vi "Calibration and Update Routine.vi"(8 "simTC Channels":dbl[](array[numeric])=[102.0], 9 "Cal Channels":dbl[](array[numeric])=[25.0, 0.0, 703.6], 10 "TC Update State":T1=enum."Update", 11 "RT Configuration Data":T2={"Current Task"="", "Voltage Task"="", "FIFO Sort Key"=[], "Cal Channel Indicies"=[0, 255, 255, 255, 255, 255, 255, 255], "Current Initial Values"=[], "Voltage Initial Values"=[], "TC Channel Config"=[{"Thermocouple Type"=0, "Temperature Units"=0}], "TC Update Period"=0.0, "Voltage Divider Ratio"=0.099, "Samples To Collect"=25.0, "Temperature Units"=0, "Cal Settling Time"=1.0, "Cal Types"=[0]} {"Cal Types" items=["J", "K", "T", "E", "N", "B", "R", "S"]; "Temperature Units" items=["Celcius", "Fahrenheit", "Kelvin", "Rankine"]; "TC Channel Config"."Temperature Units" items=["Celcius", "Fahrenheit", "Kelvin", "Rankine", "Volts"]; "TC Channel Config"."Thermocouple Type" items=["J", "K", "T", "E", "N", "B", "R", "S", "Raw Voltage"]}) -> (1 "Cal Valid?":bool, 2 "Error":dbl[](array[numeric])=[-2.86286859433152], 3 "Voltages to Output":dbl[](array[numeric])=[0.0003896684])   [LabVIEW 2011, in "Simulated Thermocouple Custom Device.lvlib"]
uses:
  Simulated Thermocouple Custom Device.lvlib
  RT Config Data.ctl
  TC Channel Config Data.ctl
  TC Selector.ctl
  TC Unit Selector.ctl
  RT TC Update State.ctl
panel:
  out "Desired temperatures to output (for debug)":dbl[](array[numeric])
  out "Reset Cal Flag":bool=TRUE
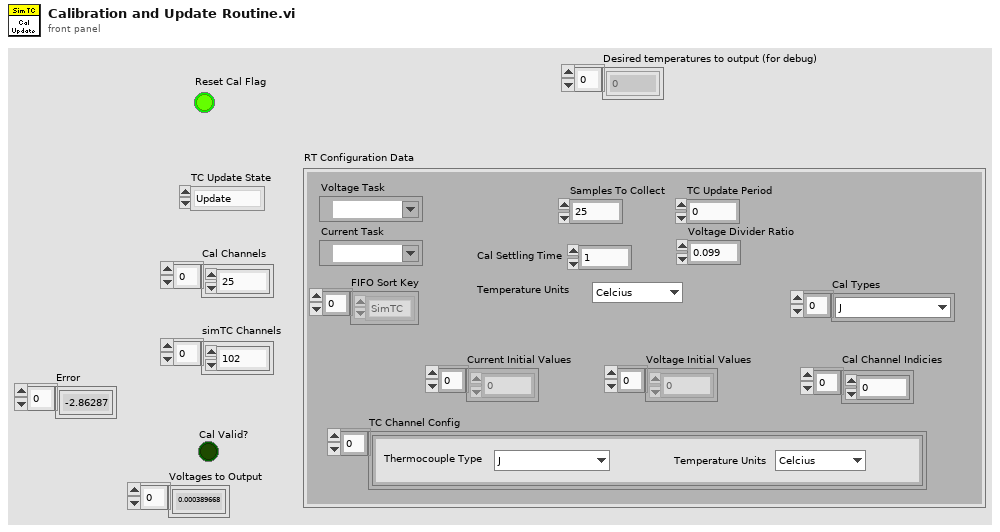
[diagram p1: front panel]
types:
  T1 = typedef "Simulated Thermocouple Custom Device.lvlib/RT TC Update State.ctl" = enum16{"Init", "Calibrate", "Update", "Idle"}
  T2 = typedef "Simulated Thermocouple Custom Device.lvlib/RT Config Data.ctl" = cluster{"Current Task":refnum<k21>, "Voltage Task":refnum<k21>, "FIFO Sort Key":enum16{"SimTC", "Calibration", "VO", "CO"}[], "Cal Channel Indicies":i32[], "Current Initial Values":dbl[], "Voltage Initial Values":dbl[], "TC Channel Config":T3[], "TC Update Period":dbl, "Voltage Divider Ratio":dbl, "Samples To Collect":dbl, "Temperature Units":T5, "Cal Settling Time":dbl, "Cal Types":T4[]}
  T3 = typedef "Simulated Thermocouple Custom Device.lvlib/TC Channel Config Data.ctl" = cluster{"Thermocouple Type":T4, "Temperature Units":T5}
  T4 = typedef "Simulated Thermocouple Custom Device.lvlib/TC Selector.ctl" = u16
  T5 = typedef "Simulated Thermocouple Custom Device.lvlib/TC Unit Selector.ctl" = u16
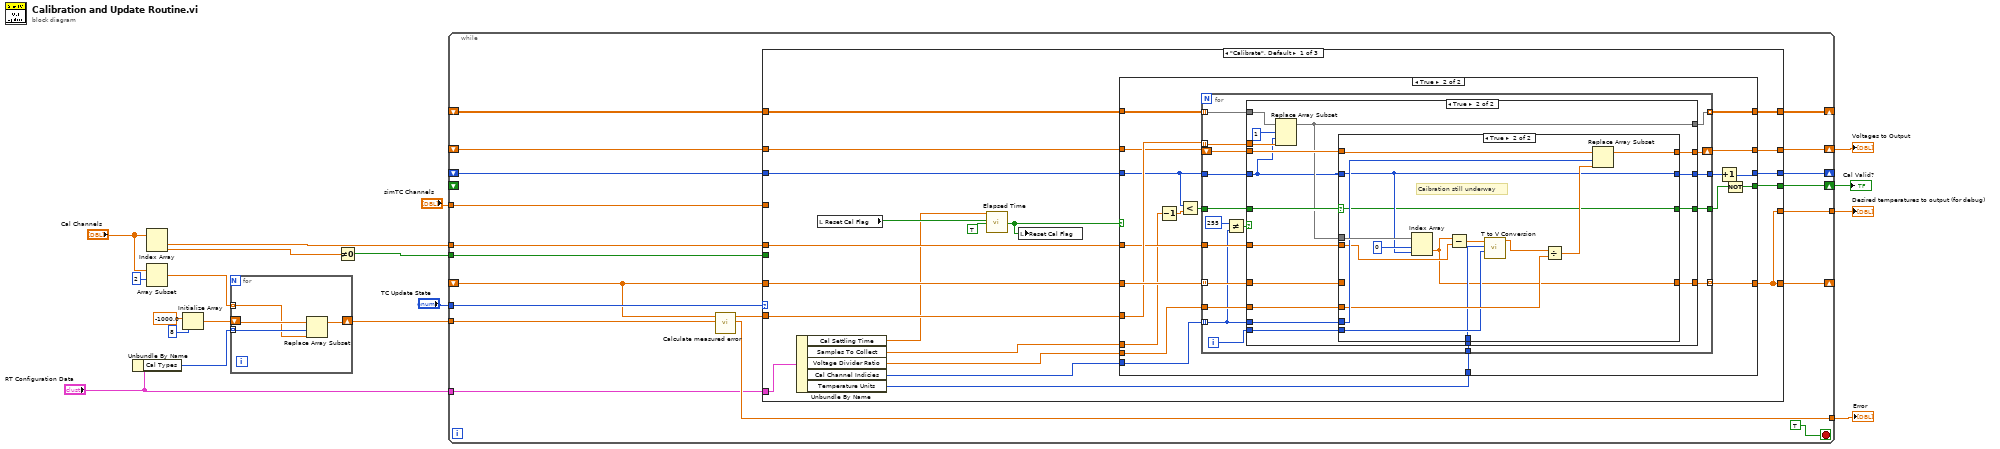
[diagram p0: block diagram]
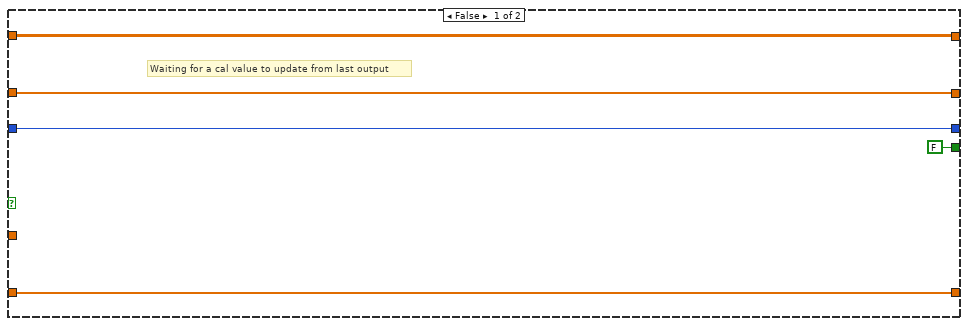
[diagram p2: hidden frame]
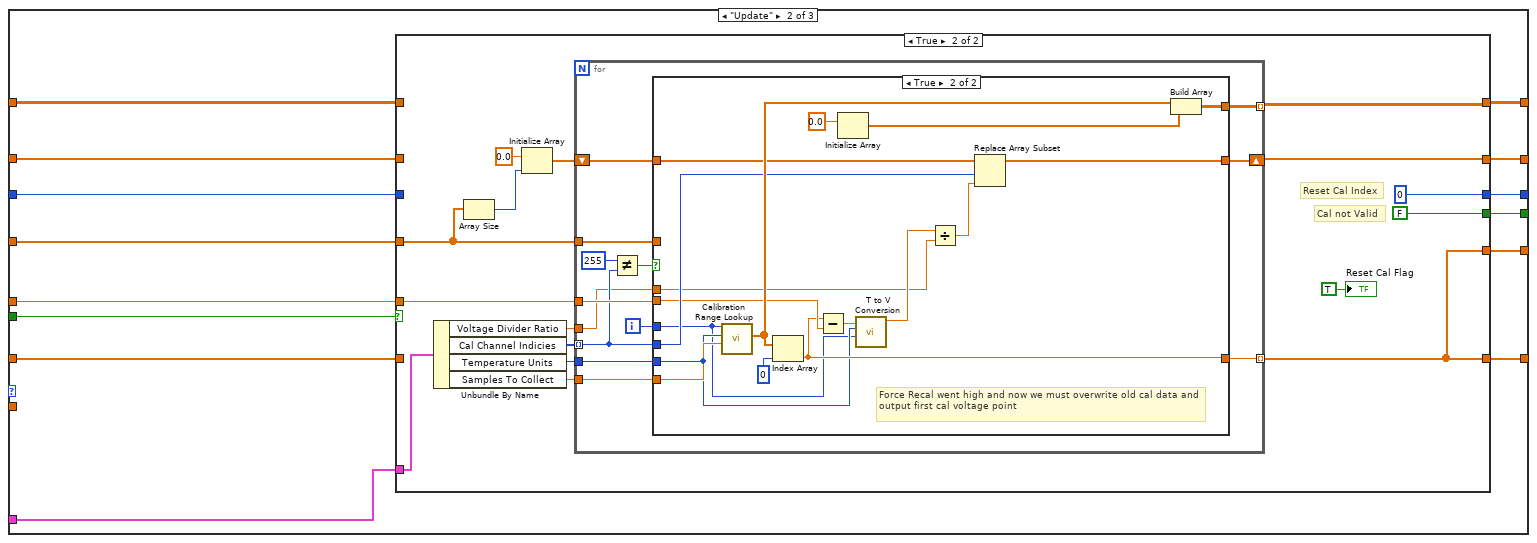
[diagram p5: hidden frame]
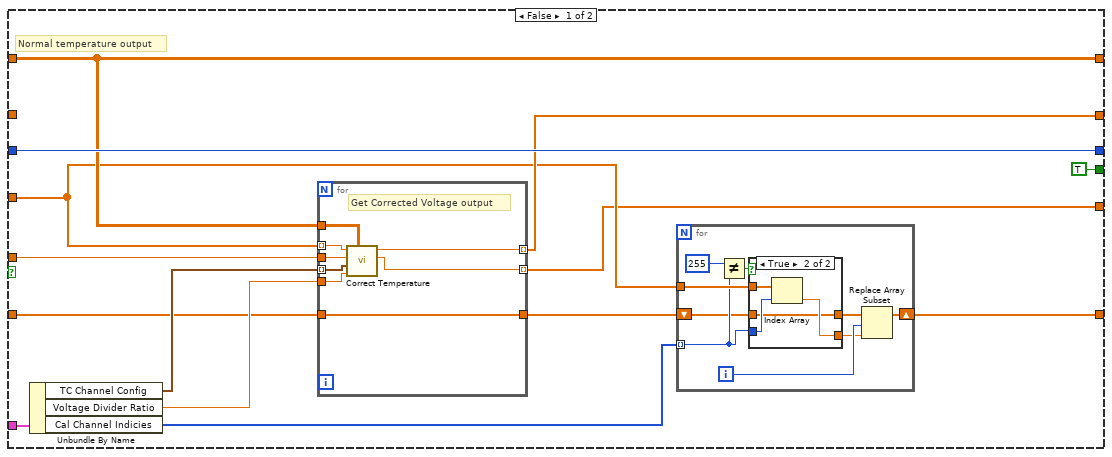
[diagram p6: hidden frame]
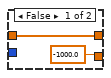
[diagram p7: hidden frame]
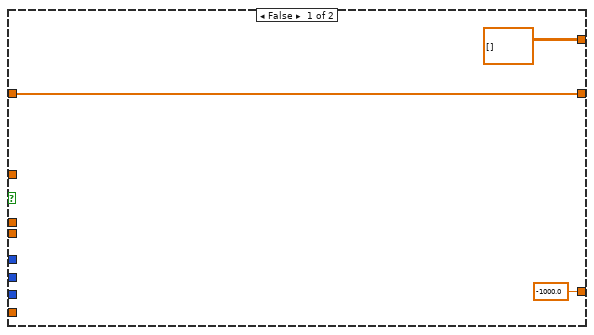
[diagram p8: hidden frame]
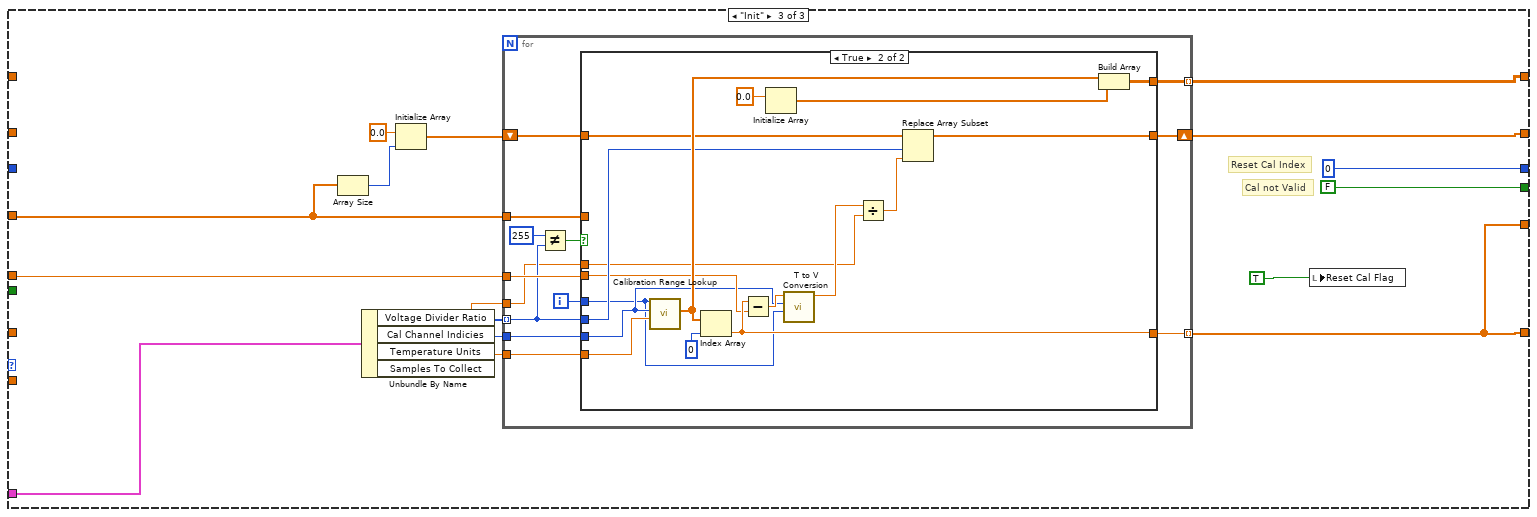
[diagram p9: hidden frame]
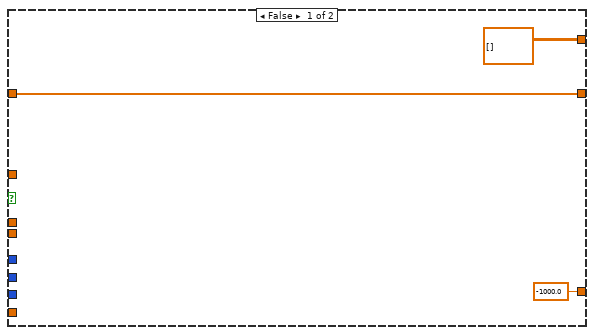
[diagram p10: hidden frame]
diagram:
  n1 = Unbundle By Name("RT Configuration Data") -> ("Cal Types"=w5:T4[])
  n2 = Index Array(array="Cal Channels") -> (element #1=w13:dbl, element #2=w12:dbl)  [unwired: 2 in]
  n3 = Array Subset(array="Cal Channels", index=2) -> (w9:dbl[])  [unwired: 1 in]
  n4 = Initialize Array(-1000.0 ("element"), 8 ("dimension size")) -> (w6:dbl[])
  n5 = for {
    tunnel: w9 -> [w19] mode=indexing
    shift-right: [w22] -> w4
    shift-left: w6 -> [w21]
    tunnel: w5 -> [w20] mode=indexing
    n6 = Replace Array Subset(array=w21, new element=w19, index=w20) -> (w22:dbl[])
  }
  n7 = Not Equal To 0?(x=w12) -> (x != 0?=w17:bool)
  n8 = while {
    tunnel: "TC Update State" -> [w40]
    tunnel: w4 -> [w26]
    tunnel: w13 -> [w28]
    tunnel: w17 -> [w37]
    shift-right: [w29] -> _
    shift-left: _ -> [w24]
    tunnel: "RT Configuration Data" -> [w30]
    shift-right: [w39] -> _
    shift-left: _ -> [w25]
    tunnel: "simTC Channels" -> [w38]
    shift-right: [w31] -> w2
    shift-left: _ -> [w34]
    tunnel: [w32] -> w15
    shift-right: [w36] -> _
    shift-left: _ -> [w27]
    shift-right: [w35] -> w14
    shift-left: _ -> [_]
    tunnel: [w23] -> w3
    stop <- TRUE stop-if-true
    n9 = call "Calculate measured error.vi"("> Cal Channel Value >"=w26, "Last Cal Channel Voltage Outputted"=w24) -> ("Error"=w32:dbl[], "Measured-Desired"=w33:dbl[])  [unwired: 8 in]
    n10 = case shown="\"Calibrate\", Default" w40 {
      tunnel: [w60 w158 w254] -> w39
      tunnel: w38 -> [_ w148 w245]
      tunnel: w25 -> [w61 w157 _]
      tunnel: w28 -> [w55 w156 w255]
      tunnel: w37 -> [_ w155 _]
      tunnel: w27 -> [w47 w152 _]
      tunnel: w33 -> [w58 _ _]
      tunnel: w24 -> [w46 w146 _]
      tunnel: [w59 w153 0] -> w36
      tunnel: [w57 w154 FALSE] -> w35
      tunnel: w34 -> [w56 w151 _]
      tunnel: [w48 w150 w253] -> w31
      tunnel: w30 -> [w51 w149 w256]
      tunnel: [w43 w147 w249] -> w29
      tunnel: [w43 w145 w249] -> w23
      frame "Calibrate", Default {
        n11 = Unbundle By Name(w51) -> ("Cal Settling Time"=w45:dbl, "Samples To Collect"=w50:dbl, "Voltage Divider Ratio"=w49:dbl, "Cal Channel Indicies"=w42:i32[], "Temperature Units"=w44:T5)
        n12 = local read "Reset Cal Flag"() -> (w53:bool)
        n13 = call "Elapsed Time"("Time Target (s)"=w45, "Reset"=w53, "Auto Reset"=TRUE) -> ("Time has Elapsed"=w52:bool)  [unwired: 9 in, 7 out]
        n14 = local write "Reset Cal Flag"(w52) -> ()
        n15 = case shown="True" w52 {
          tunnel: w61 -> [w65 w85]
          tunnel: [w65 w76] -> w60
          tunnel: w47 -> [w64 w77]
          tunnel: w46 -> [w62 w83]
          tunnel: [w64 w69] -> w59
          tunnel: w58 -> [_ w82]
          tunnel: [FALSE w68] -> w57
          tunnel: [w66 w80] -> w48
          tunnel: w56 -> [w66 w79]
          tunnel: w55 -> [_ w78]
          tunnel: w50 -> [_ w75]
          tunnel: w42 -> [_ w74]
          tunnel: w49 -> [_ w73]
          tunnel: [w62 w72] -> w43
          tunnel: w44 -> [_ w71]
          frame False {
            # "Waiting for a cal value to update from last output"
          }
          frame True {
            n16 = Decrement(x=w75) -> (x-1=w81:dbl)
            n17 = Less?(x=w77, y=w81) -> (x < y?=w84:bool)
            n18 = for {
              tunnel: w85 -> [w103] mode=indexing
              tunnel: w84 -> [w102]
              tunnel: [w101] -> w70
              tunnel: w83 -> [w100] mode=indexing
              tunnel: w82 -> [w99] mode=indexing
              tunnel: w78 -> [w96]
              tunnel: w77 -> [w92]
              tunnel: [w95] -> w76 mode=indexing
              tunnel: w74 -> [w90] mode=indexing
              tunnel: w73 -> [w94]
              tunnel: [w93] -> w72 mode=indexing
              tunnel: w71 -> [w87]
              tunnel: [w86] -> w67
              shift-right: [w98] -> w80
              shift-left: w79 -> [w97]
              i -> [w88]
              n19 = Not Equal?(x=255, y=w90) -> (x != y?=w91:bool)
              n20 = case shown="True" w91 {
                tunnel: w103 -> [w108 w125]
                tunnel: w102 -> [w104 w124]
                tunnel: [w106 w123] -> w101
                tunnel: w100 -> [w105 w122]
                tunnel: w99 -> [_ w121]
                tunnel: [w107 w120] -> w98
                tunnel: w97 -> [w107 w119]
                tunnel: w96 -> [_ w118]
                tunnel: [w108 w117] -> w95
                tunnel: w90 -> [_ w116]
                tunnel: w94 -> [_ w115]
                tunnel: [w105 w114] -> w93
                tunnel: w92 -> [w106 w112]
                tunnel: w88 -> [_ w111]
                tunnel: w87 -> [_ w110]
                tunnel: [w104 w109] -> w86
                frame False {
                }
                frame True {
                  n21 = Replace Array Subset(array=w125, new element=w121, index (row)=1 ("disabled index (row)"), index (col)=w112) -> (w117:dbl[][])
                  n22 = case shown="True" w124 {
                    selector: w124 -> [w126 w133]
                    tunnel: w112 -> [w129 w134]
                    tunnel: [w129 w134] -> w123
                    tunnel: w122 -> [w127 _]
                    tunnel: [w128 w143] -> w120
                    tunnel: w119 -> [w128 w141]
                    tunnel: w118 -> [_ w131]
                    tunnel: w117 -> [_ w142]
                    tunnel: w116 -> [_ w140]
                    tunnel: w115 -> [_ w138]
                    tunnel: [w127 w130] -> w114
                    tunnel: w111 -> [_ w136]
                    tunnel: w110 -> [_ w135]
                    tunnel: [w126 w133] -> w109
                    frame False {
                      # "Cal is Valid"
                      # "Last Step of Calibration completed"
                    }
                    frame True {
                      # "Caibration still underway"
                      n23 = Index Array(array=w142, index (row)=0, index (col)=w134) -> (element=w130:dbl)
                      n24 = Subtract(x=w130, y=w131) -> (x-y=w132:dbl)
                      n25 = call "T to V Conversion.vi"("Thermocouple Type"=w136, "Temperature Units"=w135, "Temperature"=w132) -> ("Voltage Out"=w137:dbl)  [unwired: 8 in]
                      n26 = Divide(x=w137, y=w138) -> (x/y=w139:dbl)
                      n27 = Replace Array Subset(array=w141, new element=w139, index=w140) -> (w143:dbl[])
                    }
                  }
                }
              }
            }
            n28 = Increment(x=w70) -> (x+1=w69:i32)
            n29 = Not(x=w67) -> (.not. x?=w68:bool)
          }
        }
      }
      frame "Update" {
        n30 = case shown="True" w155 {
          tunnel: [w166 w202] -> w158
          tunnel: w157 -> [w166 _]
          tunnel: w156 -> [w172 w204]
          tunnel: [TRUE FALSE] -> w154
          tunnel: [w171 0] -> w153
          tunnel: w152 -> [w171 _]
          tunnel: w151 -> [_ _]
          tunnel: [w169 w207] -> w150
          tunnel: w149 -> [w170 w209]
          tunnel: w148 -> [w160 w199]
          tunnel: [w162 w200] -> w147
          tunnel: w146 -> [w165 _]
          tunnel: [w159 w200] -> w145
          frame False {
            # "Normal temperature output"
            n31 = Unbundle By Name(w170) -> ("TC Channel Config"=w168:T3[], "Voltage Divider Ratio"=w167:dbl, "Cal Channel Indicies"=w164:i32[])
            n32 = for {
              tunnel: [w191] -> w169 mode=indexing
              tunnel: w172 -> [w195]
              tunnel: w160 -> [w189] mode=indexing
              tunnel: w168 -> [w194] mode=indexing
              tunnel: w167 -> [w193]
              tunnel: w166 -> [w192]
              tunnel: w165 -> [w190]
              tunnel: [w190] -> w163
              tunnel: [w188] -> w159 mode=indexing
              # "Get Corrected Voltage output"
              n33 = call "Correct Temperature.vi"("Cal LUT"=w192, "Divider Ratio"=w193, "TC Channel Config"=w194, "CJC"=w195, "Rquested Output Temp"=w189) -> ("Corrected Output Temp"=w188:dbl, "Voltage Out"=w191:dbl)  [unwired: 5 in]
            }
            n34 = for {
              tunnel: w164 -> [w176] mode=indexing
              tunnel: w160 -> [w181]
              shift-right: [w180] -> w162
              shift-left: w163 -> [w174]
              i -> [w179]
              n35 = Not Equal?(x=255, y=w176) -> (x != y?=w177:bool)
              n36 = case shown="True" w177 {
                tunnel: w181 -> [_ w187]
                tunnel: w176 -> [_ w186]
                tunnel: [-1000.0 ("Corrected Output Temp") w185] -> w178
                tunnel: w174 -> [w182 w184]
                tunnel: [w182 w184] -> w173
                frame False {
                }
                frame True {
                  n37 = Index Array(array=w187, index=w186) -> (element=w185:dbl)
                }
              }
              n38 = Replace Array Subset(array=w173, new element=w178, index=w179) -> (w180:dbl[])
            }
          }
          frame True {
            # "Cal not Valid"
            # "Reset Cal Index"
            n39 = Unbundle By Name(w209) -> ("Voltage Divider Ratio"=w201:dbl, "Cal Channel Indicies"=w206:i32[], "Temperature Units"=w208:T5, "Samples To Collect"=w203:dbl)
            n40 = Array Size(array=w199) -> (size(s)=w197:i32)
            n41 = Initialize Array(0.0 ("element"), w197) -> (w198:dbl[])
            n42 = for {
              tunnel: w208 -> [w224]
              tunnel: w199 -> [w223]
              tunnel: [w221] -> w200 mode=indexing
              tunnel: w206 -> [w217] mode=indexing
              tunnel: w204 -> [w220]
              tunnel: w203 -> [w219]
              tunnel: [w214] -> w202 mode=indexing
              tunnel: w201 -> [w212]
              shift-right: [w222] -> w207
              shift-left: w198 -> [w213]
              i -> [w215]
              n43 = Not Equal?(x=255, y=w217) -> (x != y?=w218:bool)
              n44 = case shown="True" w218 {
                tunnel: w224 -> [_ w229]
                tunnel: w223 -> [_ _]
                tunnel: [w226 w240] -> w222
                tunnel: [-1000.0 w230] -> w221
                tunnel: w217 -> [_ w237]
                tunnel: w220 -> [_ w231]
                tunnel: w219 -> [_ w238]
                tunnel: w215 -> [_ w228]
                tunnel: [dbl[][] [] w236] -> w214
                tunnel: w213 -> [w226 w235]
                tunnel: w212 -> [_ w233]
                frame False {
                }
                frame True {
                  # "Force Recal went high and now we must overwrite old cal data and output first cal voltage point"
                  n45 = call "Calibration Range Lookup.vi"("Samples To Collect"=w238, "Temperature Units"=w229, "Cal Channel TC Type"=w228) -> ("X-axis Values"=w243:dbl[])  [unwired: 8 in]
                  n46 = Index Array(array=w243, index=0) -> (element=w230:dbl)
                  n47 = Subtract(x=w230, y=w231) -> (x-y=w232:dbl)
                  n48 = Initialize Array(0.0 ("element")) -> (w239:dbl[])  [unwired: 1 in]
                  n49 = call "T to V Conversion.vi"("Thermocouple Type"=w228, "Temperature Units"=w229, "Temperature"=w232) -> ("Voltage Out"=w234:dbl)  [unwired: 8 in]
                  n50 = Divide(x=w234, y=w233) -> (x/y=w241:dbl)
                  n51 = Replace Array Subset(array=w235, new element=w241, index=w237) -> (w240:dbl[])
                  n52 = Build Array(w243, w239) -> (w236:dbl[][])
                }
              }
            }
            "Reset Cal Flag" <- TRUE ("Reset For Calibration")
          }
        }
      }
      frame "Init" {
        # "Cal not Valid"
        # "Reset Cal Index"
        n53 = Array Size(array=w245) -> (size(s)=w248:i32)
        n54 = Unbundle By Name(w256) -> ("Voltage Divider Ratio"=w257:dbl, "Cal Channel Indicies"=w259:i32[], "Temperature Units"=w260:T5, "Samples To Collect"=w258:dbl)
        n55 = Initialize Array(0.0 ("element"), w248) -> (w246:dbl[])
        n56 = for {
          tunnel: w260 -> [w273]
          tunnel: w245 -> [w272]
          tunnel: [w270] -> w249 mode=indexing
          tunnel: w259 -> [w266] mode=indexing
          tunnel: w255 -> [w269]
          tunnel: w258 -> [w268]
          tunnel: [w263] -> w254 mode=indexing
          tunnel: w257 -> [w261]
          shift-right: [w271] -> w253
          shift-left: w246 -> [w262]
          i -> [w264]
          n57 = Not Equal?(x=255, y=w266) -> (x != y?=w267:bool)
          n58 = case shown="True" w267 {
            tunnel: w273 -> [_ w278]
            tunnel: w272 -> [_ _]
            tunnel: [w275 w289] -> w271
            tunnel: [-1000.0 w280] -> w270
            tunnel: w266 -> [_ w286]
            tunnel: w269 -> [_ w279]
            tunnel: w268 -> [_ w287]
            tunnel: w264 -> [_ w277]
            tunnel: [dbl[][] [] w285] -> w263
            tunnel: w262 -> [w275 w284]
            tunnel: w261 -> [_ w282]
            frame False {
            }
            frame True {
              n59 = call "Calibration Range Lookup.vi"("Samples To Collect"=w287, "Temperature Units"=w278, "Cal Channel TC Type"=w277) -> ("X-axis Values"=w292:dbl[])  [unwired: 8 in]
              n60 = Index Array(array=w292, index=0) -> (element=w280:dbl)
              n61 = Subtract(x=w280, y=w279) -> (x-y=w281:dbl)
              n62 = Initialize Array(0.0 ("element")) -> (w288:dbl[])  [unwired: 1 in]
              n63 = call "T to V Conversion.vi"("Thermocouple Type"=w277, "Temperature Units"=w278, "Temperature"=w281) -> ("Voltage Out"=w283:dbl)  [unwired: 8 in]
              n64 = Divide(x=w283, y=w282) -> (x/y=w290:dbl)
              n65 = Replace Array Subset(array=w284, new element=w290, index=w286) -> (w289:dbl[])
              n66 = Build Array(w292, w288) -> (w285:dbl[][])
            }
          }
        }
        n67 = local write "Reset Cal Flag"(TRUE ("Reset For Calibration")) -> ()
      }
    }
  }
  "Error" <- w15
  "Voltages to Output" <- w2
  "Cal Valid?" <- w14
  "Desired temperatures to output (for debug)" <- w3
